vi "testExtractTopicName.vi"(8 "error in (no error)":errorcluster) -> (0 "error out":errorcluster)   [LabVIEW 2018]
uses:
  SALTypeGenerator/Module/Module.lvclass
  SALTypeGenerator/Module/Module.lvclass/Module.ctl
  <vilib>/addons/_JKI Toolkits/Caraya/classes/Assert/Assert Equal Value_Variant.vi
  <vilib>/addons/_JKI Toolkits/Caraya/classes/Test/Test.lvclass
  <vilib>/addons/_JKI Toolkits/Caraya/classes/Assert/Assert.lvclass
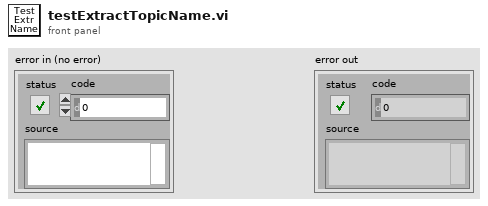
[diagram p1: front panel]
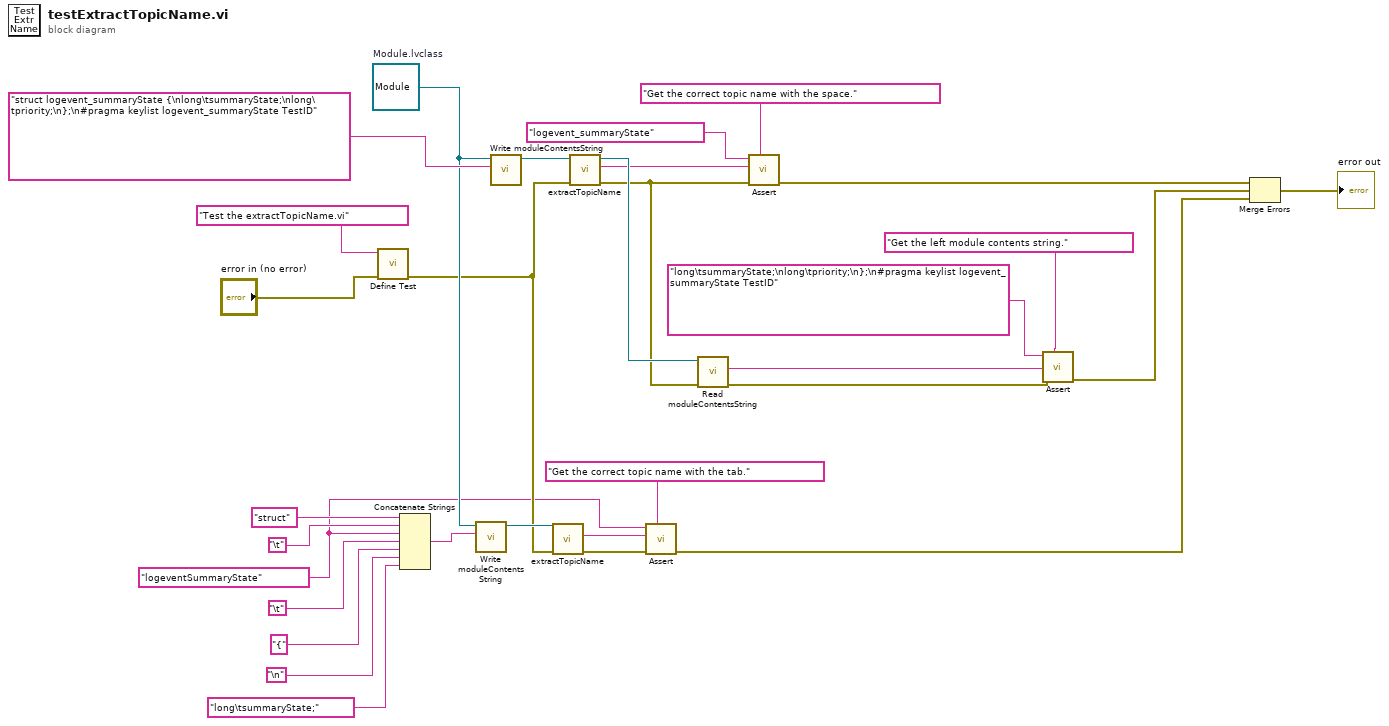
[diagram p0: block diagram]
diagram:
  w5 = "logeventSummaryState"
  w10 = refnum<class "Module.lvclass"> refnum  # Module.lvclass
  n1 = call <vilib>:"Define Test.vi"("error in (no error)"="error in (no error)", "Label (VI Title)"="Test the extractTopicName.vi") -> ("error out"=w8:errorcluster)  [unwired: 9 in]
  n2 = Concatenate Strings("struct", "\t", w5, "\t", "{", "\n", "long\tsummaryState;" ("string")) -> (w11:string)
  n3 = call "Write moduleContentsString.vi"("moduleContentsString"=w11, "Module in"=w10) -> ("Module out"=w9:refnum<class "Module.lvclass">)  [unwired: 9 in]
  n4 = call "Write moduleContentsString.vi"("moduleContentsString"="struct logevent_summaryState {\nlong\tsummaryState;\nlong\tpriority;\n};\n#pragma keylist logevent_summaryState TestID", "Module in"=w10) -> ("Module out"=w31:refnum<class "Module.lvclass">)  [unwired: 9 in]
  n5 = call "extractTopicName.vi"("error in (no error)"=w8, "Module in"=w9) -> ("error out"=w7:errorcluster, "topicName"=w6:string)  [unwired: 7 in, 1 out]
  n6 = call "extractTopicName.vi"("error in (no error)"=w8, "Module in"=w31) -> ("error out"=w26:errorcluster, "topicName"=w25:string, "Module out"=w30:refnum<class "Module.lvclass">)  [unwired: 7 in]
  n7 = call-poly <vilib>:"Assert.vi"("Label"="Get the correct topic name with the tab.", "error in (no error)"=w7, "Y"=w6, "X"=w5) -> ("error out"=w3:errorcluster)  [unwired: 7 in]
  n8 = call "Read moduleContentsString.vi"("error in (no error)"=w26, "Module in"=w30) -> ("error out"=w22:errorcluster, "moduleContentsString"=w21:string)  [unwired: 7 in, 1 out]
  n9 = call-poly <vilib>:"Assert.vi"("Label"="Get the correct topic name with the space.", "error in (no error)"=w26, "Y"=w25, "X"="logevent_summaryState") -> ("error out"=w18:errorcluster)  [unwired: 7 in]
  n10 = call-poly <vilib>:"Assert.vi"("Label"="Get the left module contents string.", "error in (no error)"=w22, "Y"=w21, "X"="long\tsummaryState;\nlong\tpriority;\n};\n#pragma keylist logevent_summaryState TestID") -> ("error out"=w17:errorcluster)  [unwired: 7 in]
  n11 = Merge Errors(w18, w17, w3) -> (→"error out":errorcluster)
